vi "Transfer Group.Is Active.vi"(10 "cycle count":u64=1, 11 "Transfer Group in":refnum<class "Transfer Group.lvclass">) -> (2 "active this cycle?":bool, 3 "Transfer Group out":refnum<class "Transfer Group.lvclass">)   [LabVIEW 2017, in "DSF Core.lvlib" / "Transfer Group.lvclass"]
uses:
  Transfer Group.lvclass
  Transfer Group.lvclass/Transfer Group.ctl
  Timing/Timing.lvclass/Timing.ctl
  Timing/Get Decimation.vi
  Timing/Get Offset.vi
  Timing/Timing.lvclass
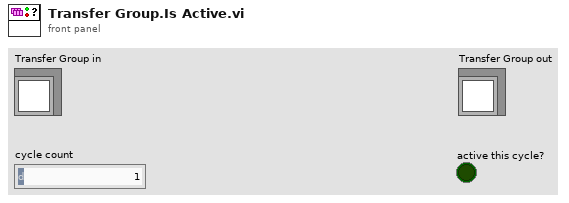
[diagram p1: front panel]
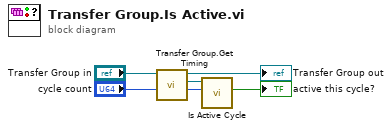
[diagram p0: block diagram]
diagram:
  n1 = call "Transfer Group.Get Timing.vi"("Transfer Group in"="Transfer Group in") -> ("Timing"=w4:refnum<class "Timing.lvclass">, "Transfer Group out"=→"Transfer Group out":refnum<class "Transfer Group.lvclass">)  [unwired: 9 in]
  n2 = call "Is Active Cycle.vi"("iteration"="cycle count", "Timing in"=w4) -> ("active?"=→"active this cycle?":bool)  [unwired: 8 in, 1 out]
